vi "UT_Waterfall.vi"(10 "Waveform 2D In":T1(array[cluster]), 11 "Waterfall Offset":dbl=0.1) -> (2 "Graph":T1(graph)=[{"relativeInitialX"=8.61e-06, "xIncrement"=1e-08, "measWfm"=[0.001229284415, 0.000531437126, 3.3874462e-05, -0.000262757317, -0.000843136503, -0.001442352086, -0.001307764221, -0.000771927918, -0.000371442851, 0.000414477841, 0.001937090225, 0.003518533596, 0.004546074676, 0.003762970376, -0.004259295561, -0.02497045342, -0.046262873477, -0.031038040104, 0.04908052842, 0.15361398773, 0.175964427137, 0.036062506373, -0.218876584634, -0.39105984646, -0.289618582995, 0.057799753479, 0.405506738709, 0.489887339955, 0.249687387616, -0.125686036106, -0.369324899822, -0.351797544271, -0.146225843205, 0.075461074684, 0.1851618293, 0.162830744515, 0.068689117359, -0.020603397133, -0.06017529904, -0.049854322594, -0.016333562471, 0.012084053874, 0.020872433594, 0.011077563012, -0.007409282979, -0.021880102361, -0.021219837949, -0.001976867848, 0.025698637853, 0.040994274431, 0.02782932291, -0.008795481912, -0.043822447558, -0.052095170143, -0.028304342641, 0.010155044803, 0.038718251647, 0.043655660529, 0.027425970176, 0.002402566994, -0.018705459061, -0.028141958537, -0.02339687303, -0.007926334944, 0.008977714371, 0.017310120047, 0.013424324003, 0.002241532571, -0.007778876073, -0.011361232689, -0.009040759694, -0.003461049461, 0.004755231013, 0.014231401436, 0.019339013738, 0.013293688103, -0.004261636478, -0.023251418347, -0.02979530714, -0.018175200525, 0.004283292349, 0.023107881058, 0.027393277423, 0.017050152868, 0.000631130412, -0.013002595416, -0.019435100192, -0.017638825872, -0.007889835918, 0.007543876091, 0.021512452292, 0.02368276486, 0.00938255249, -0.013767975985, -0.029789714977, -0.026753068415, -0.006652195363, 0.016720516212, 0.029103108037, 0.025345065159, 0.009757959295, -0.008809061368, -0.021889515976, -0.0245565713, -0.01584607994, 0.00013470681, 0.014881949842, 0.02066451973, 0.01531767711, 0.003481997139, -0.006951780004, -0.010814685245, -0.008748755867, -0.004318584634, 0.000332428544, 0.00403344523, 0.005028146099, 0.002699889114, -0.001098666986, -0.003676539341, -0.003893919854, -0.002247586025, 0.000462604981, 0.003425489866, 0.005944032857, 0.006961374095, 0.004620429152, -0.001873108371, -0.009776610996, -0.013130930041, -0.007852488221, 0.002998441254, 0.011649354388, 0.012345454441, 0.005442026149, -0.003045044174, -0.007146808097, -0.005933325513, -0.002355210962, 0.000486440322, 0.00145658781, 0.001228933151, 0.000690244803, -0.00018895918, -0.001223393833, -0.001030319571, 0.000827632335, 0.002582253067, 0.002688164246, 0.001524506133, 0.000253589348, -0.000659000363, -0.001669901954, -0.003205996288, -0.00447804353, -0.003500995549, 0.000557212705, 0.005609829375, 0.00782439829, 0.004686567793, -0.001762264188, -0.00679924282, -0.007510820459, -0.003702014629, 0.002672274903, 0.007942356876, 0.008150038713, 0.002511544297, -0.004946106109, -0.008958686915, -0.00743633888, -0.001986194597, 0.004154525654, 0.007581091102, 0.006666021023, 0.002942943935, -0.000938407687, -0.003685212876, -0.005343487441, -0.005604621435, -0.003282403705, 0.001447903172, 0.005944497031, 0.006936815024, 0.003267718408, -0.002372135952, -0.005619322164, -0.004617028226, -0.001055801449, 0.00206697821, 0.003165425539, 0.002563850732, 0.001088148398, -0.000685939699, -0.002333598865, -0.00286658691, -0.001420307517, 0.001172603982, 0.003048681733, 0.002836818095, 0.000783075614, -0.001463005959, -0.002619422961, -0.002665753539, -0.001870911336, -0.000267591391, 0.001988624698, 0.004191435598, 0.004435725075, 0.001364485544, -0.003151237708, -0.00546650415, -0.004187041276, -0.000775831695, 0.002779680332, 0.00466277436, 0.003752202708, 0.00064037598, -0.002639968168, -0.00408340386, -0.002991606311, -0.000145261242, 0.002414024649, 0.00317583172, 0.002313228274, 0.000589339893, -0.001123389242, -0.002221502611, -0.002509017937, -0.001932191189, -0.000749081053, 0.000711149352, 0.002172197353, 0.003242534733, 0.003167262714, 0.001368580601, -0.001766867708, -0.004632718725, -0.004729816316, -0.001448662144, 0.002538444402, 0.004231721426, 0.003188948149, 0.001025872291, -0.000830015105, -0.002031367206, -0.002589059119, -0.00217349028, -0.000737239122, 0.001157079026, 0.002623582993, 0.002647122268, 0.001114331658, -0.000868528191, -0.002227482752, -0.002724396411, -0.002263491863, -0.000486850693, 0.002045755539, 0.003724103019, 0.003254439413, 0.000680982217, -0.002161240044, -0.003227561333, -0.002185806114, -0.000218008055, 0.001234752643, 0.001720310862, 0.001592579417, 0.000765235298, -0.00073528965, -0.002031014293, -0.002077452044, -0.000334245449, 0.002268391708, 0.003393655312, 0.001278216118, -0.002496109203, -0.004249862588, -0.002565794648, 0.000795307006, 0.002910022142, 0.002967234426, 0.002194157911, 0.001193536387, -0.000194148907, -0.001975540423, -0.003390640925, -0.003620971043, -0.002737737017, -0.00108340157, 0.00147595603, 0.004663592221, 0.007177747669, 0.00715133456, 0.002862424818, -0.004664133338, -0.010645824776, -0.010804265054, -0.004954474501, 0.003269720209, 0.008906048969, 0.009187289445, 0.004677680584, -0.001498623569, -0.005436027894, -0.00538169373, -0.002795394164, -2.9810499e-05, 0.002059367373, 0.003202580309, 0.002815595461, 0.000854512165, -0.001435171814, -0.002464195961, -0.002260253376, -0.001539562146, -0.00035054247, 0.001292648569]}, ...(2 in all)] caption="A - Scan Graph")   [LabVIEW 2012]
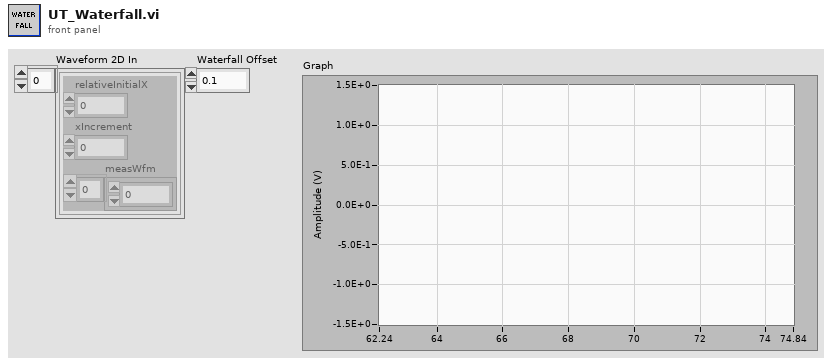
[diagram p1: front panel]
types:
  T1 = cluster{"relativeInitialX":dbl, "xIncrement":dbl, "measWfm":dbl[]}[]
  T2 = cluster{"relativeInitialX":dbl, "xIncrement":dbl, "measWfm":dbl[]}
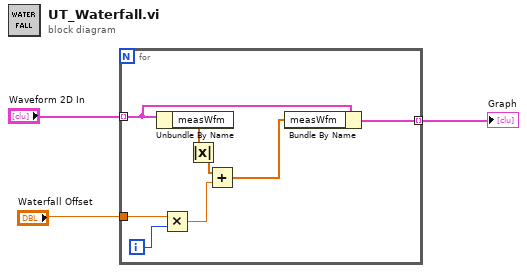
[diagram p0: block diagram]
diagram:
  n1 = for {
    tunnel: "Waveform 2D In" -> [w8] mode=indexing
    tunnel: "Waterfall Offset" -> [w11]
    tunnel: [w6] -> w1 mode=indexing
    i -> [w5]
    n2 = Unbundle By Name(w8) -> ("measWfm"=w9:dbl[])
    n3 = Multiply(x=w11, y=w5) -> (x*y=w10:dbl)
    n4 = Absolute Value(x=w9) -> (abs(x)=w4:dbl[])
    n5 = Add(x=w4, y=w10) -> (x+y=w7:dbl[])
    n6 = Bundle By Name(cluster=w8, "measWfm"=w7) -> (w6:T2)
  }
  "Graph" <- w1
